vi "ArrayToString.vi"(1 "Format":string, 2 "Input 1D array":dbl[](array[numeric])) -> (7 "Output 1D array":string[](array[string]))   [LabVIEW 2015]
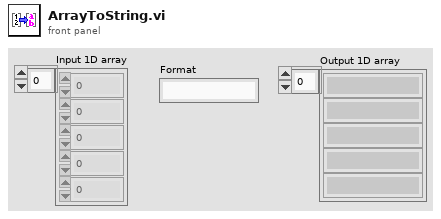
[diagram p1: front panel]
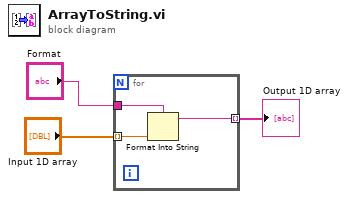
[diagram p0: block diagram]
diagram:
  n1 = for {
    tunnel: "Input 1D array" -> [w6] mode=indexing
    tunnel: "Format" -> [w5]
    tunnel: [w4] -> w2 mode=indexing
    n2 = Format Into String(format string=w5, w6) -> (resulting string=w4:string)  [unwired: 2 in, 1 out]
  }
  "Output 1D array" <- w2
